vi "GetPrefsAfterInitDone.vi"(2 "error in (no error)":errorcluster) -> (0 "error out":errorcluster, 1 "Preferences out":refnum<class "SetListPrefs.lvclass">)   [LabVIEW 2013, in "SetListPrefs.lvclass"]
uses:
  SetListPrefs.lvclass
  Globals/PrefsGlobal.vi
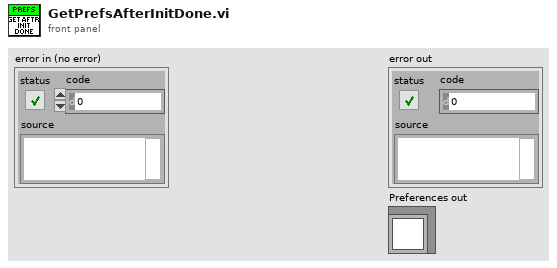
[diagram p1: front panel]
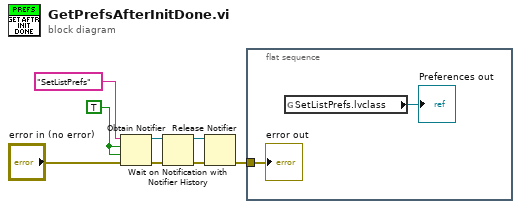
[diagram p0: block diagram]
diagram:
  w7 = TRUE
  n1 = Obtain Notifier(name (unnamed)="SetListPrefs", notification data type=w7, create if not found? (T)=w7, error in (no error)="error in (no error)") -> (notifier out=w4:refnum<notifier>, error out=w5:errorcluster)  [unwired: 1 out]
  n2 = Wait on Notification with Notifier History(0:w4, 3:w5) -> (8:w2:refnum<notifier>, 11:w3:errorcluster)  [unwired: 2 in, 2 out]
  n3 = Release Notifier(notifier=w2, error in (no error)=w3) -> (error out=w1:errorcluster)  [unwired: 1 in, 2 out]
  n4 = flat-sequence {
    tunnel: w1 -> [w10]
    frame #0 {
      n5 = global read "PrefsGlobal.vi" "SetListPrefs.lvclass"() -> (→"Preferences out":refnum<class "SetListPrefs.lvclass">)
      "error out" <- w10
    }
  }
